vi "soundcard.vi"() -> ()   [LabVIEW 2013]
uses:
  <vilib>/sound2/lvsound2.llb/Sampling Mode.ctl
  <vilib>/sound2/lvsound2.llb/Sound Data Format.ctl
  <vilib>/sound2/lvsound2.llb/Sound Output Write (DBL Single).vi
  <vilib>/Analysis/NI_AALBase.lvlib
panel:
  in  "sound format":T1={"sample rate (S/s)"=22050.0, "number of channels"=2, "bits per sample"=16}
  in  "device ID":u32
  in  "number of samples/ch":i32=100000
  in  "sample mode":T2=1 items=["Finite Samples", "Continuous Samples"]
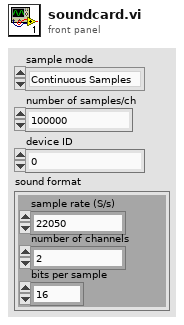
[diagram p1: front panel]
types:
  T1 = typedef "Sound Data Format.ctl" = cluster{"sample rate (S/s)":dbl, "number of channels":i32, "bits per sample":i32}
  T2 = typedef "Sampling Mode.ctl" = i32
  T3 = typedef "Sound Output Task ID.ctl" = u32
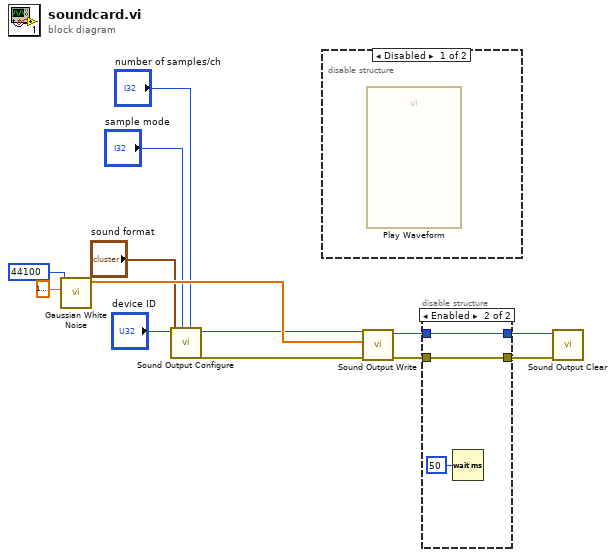
[diagram p0: block diagram]
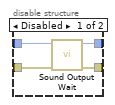
[diagram p2: hidden frame]
diagram:
  n1 = call <vilib>:"Gaussian White Noise.vi"("standard deviation"=1.0000000000000002, "samples"=44100) -> ("Gaussian noise pattern"=w11:dbl[])  [unwired: 8 in, 1 out]
  n2 = call <vilib>:"Sound Output Configure.vi"("number of samples/ch"="number of samples/ch", "sample mode"="sample mode", "sound format"="sound format", "device ID"="device ID") -> ("error out"=w2:errorcluster, "task ID"=w10:T3)  [unwired: 6 in]
  n3 = disable-structure shown="Disabled" {
    frame Disabled {
      n4 = call "Play Waveform"() -> ()  [unwired: 19 in, 1 out]
    }
    frame Enabled {
    }
  }
  n5 = call-poly <vilib>:"Sound Output Write.vi"("error in (no error)"=w2, "data"=w11, "task ID"=w10) -> ("error out"=w3:errorcluster, "task ID out"=w1:T3)  [unwired: 7 in]
  n6 = disable-structure shown="Enabled" {
    disable-tunnel: [w17 w20] -> w5
    disable-tunnel: [w16 w19] -> w4
    disable-tunnel: w3 -> [w15 w19]
    disable-tunnel: w1 -> [w14 w20]
    frame Disabled {
      n7 = call <vilib>:"Sound Output Wait.vi"("error in (no error)"=w15, "task ID"=w14) -> ("error out"=w16:errorcluster, "task ID out"=w17:T3)  [unwired: 8 in]
    }
    frame Enabled {
      n8 = Wait (ms)(milliseconds to wait=u32 50) -> ()  [unwired: 1 out]
    }
  }
  n9 = call <vilib>:"Sound Output Clear.vi"("error in (no error)"=w4, "task ID"=w5) -> ()  [unwired: 9 in, 1 out]
